vi "testRunCallsRunTest.vi"() -> (0 "error out":errorcluster)   [LabVIEW 2019, in "TestResultTest.lvlib"]
uses:
  TestResultTest.lvlib
  TestResult/TestResult.lvclass
  TestResultTestSupport/TestCaseMock/TestCaseMock.lvclass
  C:/Users/de200256/Code/LVUnit/TestCase/TestCase/TestCase.lvclass
  Assertion/Assertion.lvlib
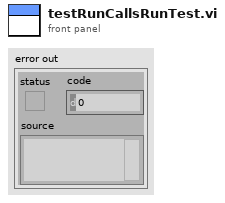
[diagram p1: front panel]
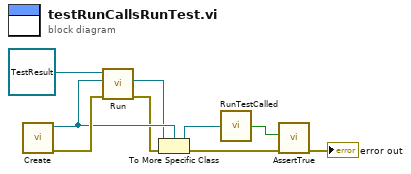
[diagram p0: block diagram]
diagram:
  n1 = call "Create.vi"() -> ("error out"=w8:errorcluster, "TestCaseMock"=w7:refnum<class "TestCaseMock.lvclass">)  [unwired: 10 in]
  n2 = call-dynamic "Run.vi"("error in (no error)"=w8, "TestCase"=w7, "TestResult in"=refnum<class "TestResult.lvclass"> refnum ("TestResult.lvclass")) -> ("error out"=w2:errorcluster, "TestCase out"=w3:refnum<class "TestCase.lvclass">)  [unwired: 6 in, 1 out]
  n3 = To More Specific Class(target class=w7, reference=w3, error in=w2) -> (specific class reference=w6:refnum<class "TestCaseMock.lvclass">, error out=w9:errorcluster)
  n4 = call "RunTestCalled.vi"("TestCaseMock In"=w6) -> ("RunTest Called"=w4:bool)
  n5 = call "AssertTrue.vi"("error in (no error)"=w9, "Condition"=w4) -> ("error out"=→"error out":errorcluster)  [unwired: 9 in]
